vi "RTS Find Earliest Start Time.vi"(8 "Error In":errorcluster, 11 "All Door Opener Ctrl":T4 {"Station 8"."Station Slide"."Chamber 1-1"."Start Time" format="%<%X\n%x>T"; "Station 8"."Station Slide"."Chamber 1-1"."End Time" format="%<%X\n%x>T"; "Station 8"."Station Slide"."Time Count (s)" format="%.2f"; "Station 8"."Station Cab"."Chamber 1-1"."Start Time" format="%<%X\n%x>T"; "Station 8"."Station Cab"."Chamber 1-1"."End Time" format="%<%X\n%x>T"; "Station 8"."Station Cab"."Time Count (s)" format="%.2f"; "Station 8"."Station Freezer"."Chamber 1-1"."Start Time" format="%<%X\n%x>T"; "Station 8"."Station Freezer"."Chamber 1-1"."End Time" format="%<%X\n%x>T"; "Station 8"."Station Freezer"."Time Count (s)" format="%.2f"; "Station 7"."Station Slide"."Chamber 1-1"."Start Time" format="%<%X\n%x>T"; "Station 7"."Station Slide"."Chamber 1-1"."End Time" format="%<%X\n%x>T"; "Station 7"."Station Slide"."Time Count (s)" format="%.2f"; "Station 7"."Station Cab"."Chamber 1-1"."Start Time" format="%<%X\n%x>T"; "Station 7"."Station Cab"."Chamber 1-1"."End Time" format="%<%X\n%x>T"; "Station 7"."Station Cab"."Time Count (s)" format="%.2f"; "Station 7"."Station Freezer"."Chamber 1-1"."Start Time" format="%<%X\n%x>T"; "Station 7"."Station Freezer"."Chamber 1-1"."End Time" format="%<%X\n%x>T"; "Station 7"."Station Freezer"."Time Count (s)" format="%.2f"; "Station 6"."Station Slide"."Chamber 1-1"."Start Time" format="%<%X\n%x>T"; "Station 6"."Station Slide"."Chamber 1-1"."End Time" format="%<%X\n%x>T"; "Station 6"."Station Slide"."Time Count (s)" format="%.2f"; "Station 6"."Station Cab"."Chamber 1-1"."Start Time" format="%<%X\n%x>T"; "Station 6"."Station Cab"."Chamber 1-1"."End Time" format="%<%X\n%x>T"; "Station 6"."Station Cab"."Time Count (s)" format="%.2f"; "Station 6"."Station Freezer"."Chamber 1-1"."Start Time" format="%<%X\n%x>T"; "Station 6"."Station Freezer"."Chamber 1-1"."End Time" format="%<%X\n%x>T"; "Station 6"."Station Freezer"."Time Count (s)" format="%.2f"; "Station 5"."Station Slide"."Chamber 1-1"."Start Time" format="%<%X\n%x>T"; "Station 5"."Station Slide"."Chamber 1-1"."End Time" format="%<%X\n%x>T"; "Station 5"."Station Slide"."Time Count (s)" format="%.2f"; "Station 5"."Station Cab"."Chamber 1-1"."Start Time" format="%<%X\n%x>T"; "Station 5"."Station Cab"."Chamber 1-1"."End Time" format="%<%X\n%x>T"; "Station 5"."Station Cab"."Time Count (s)" format="%.2f"; "Station 5"."Station Freezer"."Chamber 1-1"."Start Time" format="%<%X\n%x>T"; "Station 5"."Station Freezer"."Chamber 1-1"."End Time" format="%<%X\n%x>T"; "Station 5"."Station Freezer"."Time Count (s)" format="%.2f"; "Station 4"."Station Slide"."Chamber 1-1"."Start Time" format="%<%X\n%x>T"; "Station 4"."Station Slide"."Chamber 1-1"."End Time" format="%<%X\n%x>T"; "Station 4"."Station Slide"."Time Count (s)" format="%.2f"; "Station 4"."Station Cab"."Chamber 1-1"."Start Time" format="%<%X\n%x>T"; "Station 4"."Station Cab"."Chamber 1-1"."End Time" format="%<%X\n%x>T"; "Station 4"."Station Cab"."Time Count (s)" format="%.2f"; "Station 4"."Station Freezer"."Chamber 1-1"."Start Time" format="%<%X\n%x>T"; "Station 4"."Station Freezer"."Chamber 1-1"."End Time" format="%<%X\n%x>T"; "Station 4"."Station Freezer"."Time Count (s)" format="%.2f"; "Station 3"."Station Slide"."Chamber 1-1"."Start Time" format="%<%X\n%x>T"; "Station 3"."Station Slide"."Chamber 1-1"."End Time" format="%<%X\n%x>T"; "Station 3"."Station Slide"."Time Count (s)" format="%.2f"; "Station 3"."Station Cab"."Chamber 1-1"."Start Time" format="%<%X\n%x>T"; "Station 3"."Station Cab"."Chamber 1-1"."End Time" format="%<%X\n%x>T"; "Station 3"."Station Cab"."Time Count (s)" format="%.2f"; "Station 3"."Station Freezer"."Chamber 1-1"."Start Time" format="%<%X\n%x>T"; "Station 3"."Station Freezer"."Chamber 1-1"."End Time" format="%<%X\n%x>T"; "Station 3"."Station Freezer"."Time Count (s)" format="%.2f"; "Station 2"."Station Slide"."Chamber 1-1"."Start Time" format="%<%X\n%x>T"; "Station 2"."Station Slide"."Chamber 1-1"."End Time" format="%<%X\n%x>T"; "Station 2"."Station Slide"."Time Count (s)" format="%.2f"; "Station 2"."Station Cab"."Chamber 1-1"."Start Time" format="%<%X\n%x>T"; "Station 2"."Station Cab"."Chamber 1-1"."End Time" format="%<%X\n%x>T"; "Station 2"."Station Cab"."Time Count (s)" format="%.2f"; "Station 2"."Station Freezer"."Chamber 1-1"."Start Time" format="%<%X\n%x>T"; "Station 2"."Station Freezer"."Chamber 1-1"."End Time" format="%<%X\n%x>T"; "Station 2"."Station Freezer"."Time Count (s)" format="%.2f"; "Station 1"."Station Slide"."Chamber 1-1"."Start Time" format="%<%X\n%x>T"; "Station 1"."Station Slide"."Chamber 1-1"."End Time" format="%<%X\n%x>T"; "Station 1"."Station Slide"."Time Count (s)" format="%.2f"; "Station 1"."Station Cab"."Chamber 1-1"."Start Time" format="%<%X\n%x>T"; "Station 1"."Station Cab"."Chamber 1-1"."End Time" format="%<%X\n%x>T"; "Station 1"."Station Cab"."Time Count (s)" format="%.2f"; "Station 1"."Station Freezer"."Chamber 1-1"."Start Time" format="%<%X\n%x>T"; "Station 1"."Station Freezer"."Chamber 1-1"."End Time" format="%<%X\n%x>T"; "Station 1"."Station Freezer"."Time Count (s)" format="%.2f"}) -> (0 "Error Out":errorcluster, 2 "Index":i32, 3 "Chamber 1-1":T1={"End Time"=timestamp(0 s since 1904-01-01), "Start Time"=timestamp(0 s since 1904-01-01), "Door Opening Schedule:"={"Open Door Timer (s)"=10.0, "Delay Time (s)"=10.0, "Close Door Timer (s)"=10.0}, "Enable Door Ops"=FALSE, "Door Openings"=0, "Temp (°F)"=0.0, "Humidity (%)"=0.0, "Voltage (V)"=0.0, "Door Open Sequence:"=enum."", "Door Delay(sec)"=0.0, "Dehum (°F)"=0.0, "Cool (°F)"=0.0} {"Start Time" format="%<%X\n%x>T"; "End Time" format="%<%X\n%x>T"})   [LabVIEW 2016]
uses:
  Type Definitions/RTS All Station Door Opener Ctrl.ctl
  Type Definitions/RTS Station Relay Ops.ctl
  Type Definitions/RTS Door Opener Indicator.ctl
  Type Definitions/RTS Door Ops Client.ctl
  Type Definitions/RTS Door Opening Schedule.ctl
  Type Definitions/RTS Door Ops Sequence.ctl
panel:
  # "Chamber Conditions:"
  # "Chamber Conditions:"
  # "Chamber Conditions:"
  # "Chamber Conditions:"
  # "Chamber Conditions:"
  # "Chamber Conditions:"
  # "Chamber Conditions:"
  # "Chamber Conditions:"
  # "Chamber Conditions:"
  # "Chamber Conditions:"
  # "Chamber Conditions:"
  # "Chamber Conditions:"
  # "Chamber Conditions:"
  # "Chamber Conditions:"
  # "Chamber Conditions:"
  # "Chamber Conditions:"
  # "Chamber Conditions:"
  # "Chamber Conditions:"
  # "Chamber Conditions:"
  # "Chamber Conditions:"
  # "Chamber Conditions:"
  # "Chamber Conditions:"
  # "Chamber Conditions:"
  # "Chamber Conditions:"
  # "Chamber Conditions:"
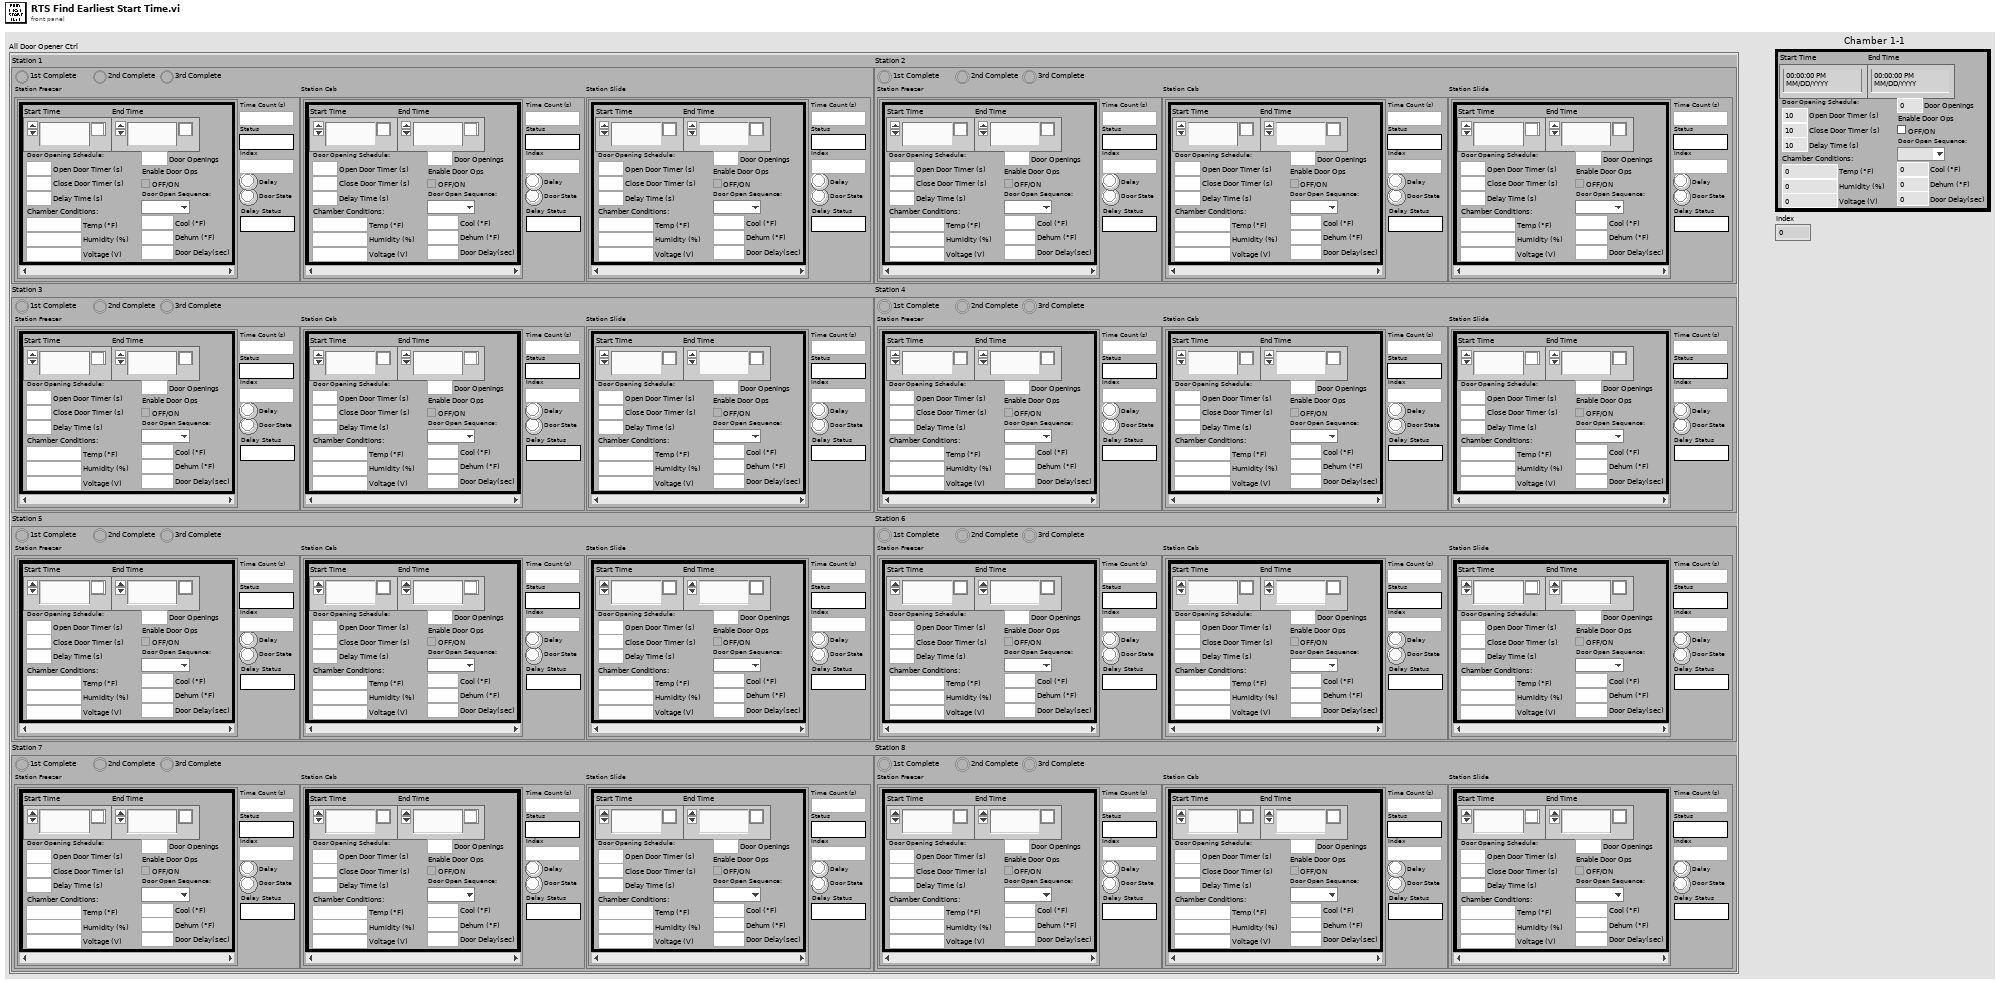
[diagram p1: front panel]
types:
  T1 = typedef "RTS Door Ops Client.ctl" = cluster{"End Time":timestamp, "Start Time":timestamp, "Door Opening Schedule:":T2, "Enable Door Ops":bool, "Door Openings":u32, "Temp (°F)":dbl, "Humidity (%)":dbl, "Voltage (V)":dbl, "Door Open Sequence:":T3, "Door Delay(sec)":dbl, "Dehum (°F)":dbl, "Cool (°F)":dbl}
  T2 = typedef "RTS Door Opening Schedule.ctl" = cluster{"Open Door Timer (s)":dbl, "Delay Time (s)":dbl, "Close Door Timer (s)":dbl}
  T3 = typedef "RTS Door Ops Sequence.ctl" = enum16{"", "1st", "2nd", "3rd"}
  T4 = typedef "RTS All Station Door Opener Ctrl.ctl" = cluster{"Station 1":T5, "Station 2":T5, "Station 3":T5, "Station 4":T5, "Station 5":T5, "Station 6":T5, "Station 7":T5, "Station 8":T5}
  T5 = typedef "RTS Station Relay Ops.ctl" = cluster{"Station Freezer":T6, "Station Cab":T6, "Station Slide":T6, "1st Complete":bool, "2nd Complete":bool, "3rd Complete":bool}
  T6 = typedef "RTS Door Opener Indicator.ctl" = cluster{"Time Count (s)":dbl, "Status":string, "Door State":bool, "Delay":bool, "Chamber 1-1":T1[], "Index":i32, "Delay Status":string}
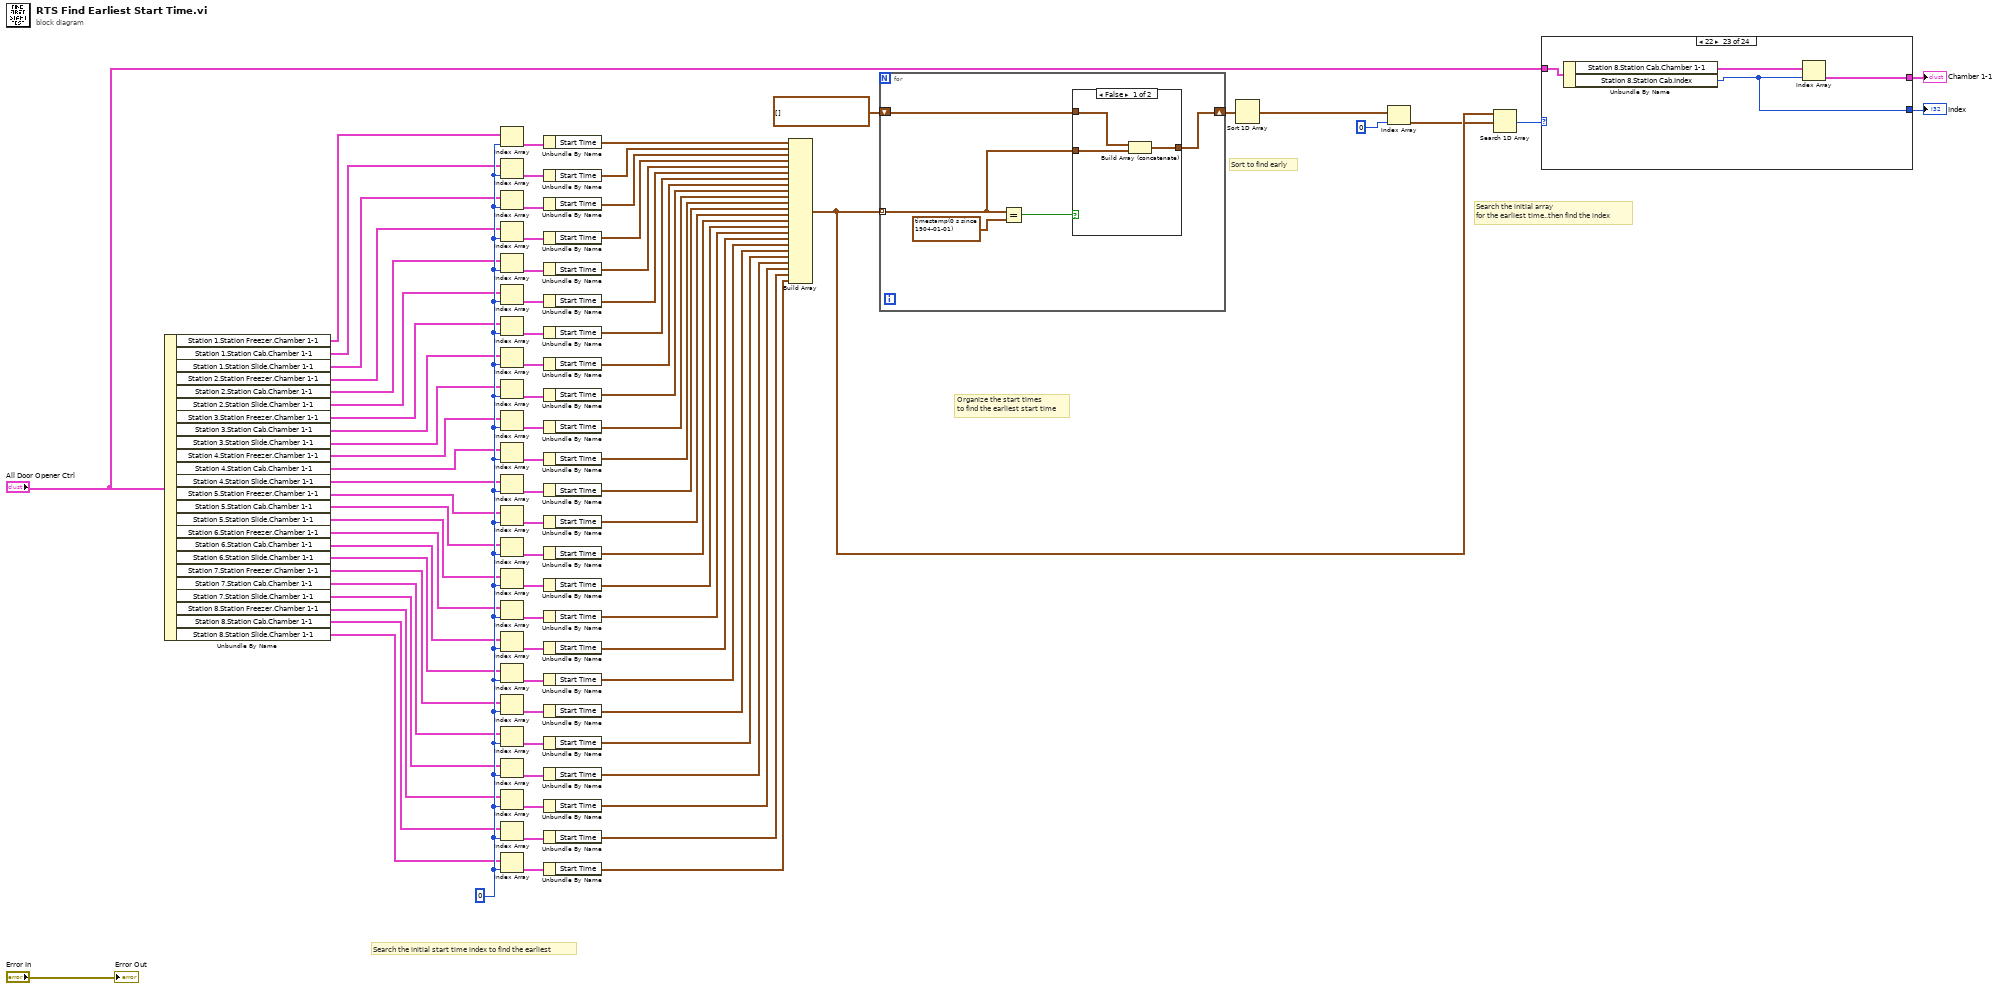
[diagram p0: block diagram]
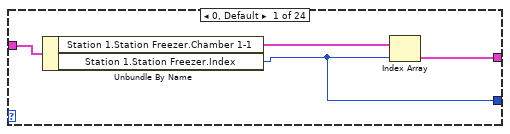
[diagram p2: hidden frame]
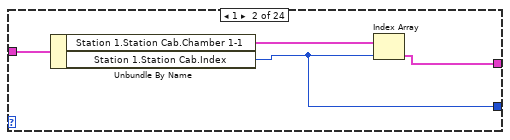
[diagram p3: hidden frame]
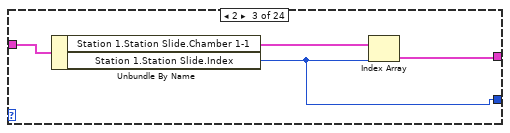
[diagram p4: hidden frame]
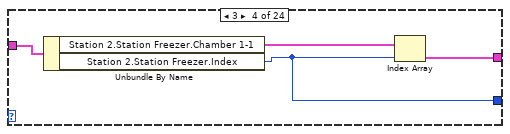
[diagram p5: hidden frame]
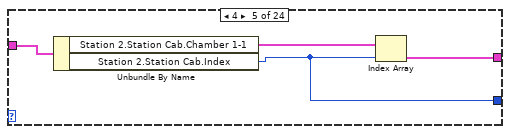
[diagram p6: hidden frame]
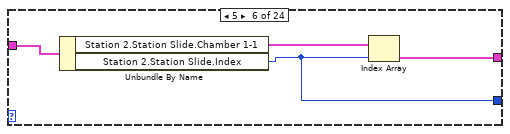
[diagram p7: hidden frame]
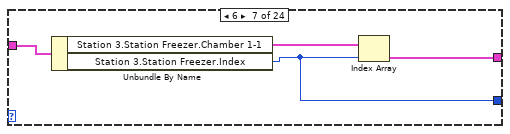
[diagram p8: hidden frame]
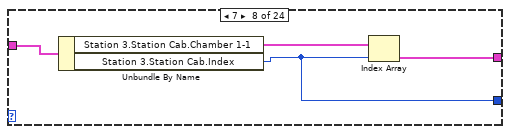
[diagram p9: hidden frame]
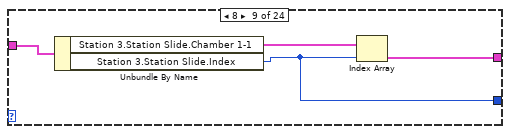
[diagram p10: hidden frame]
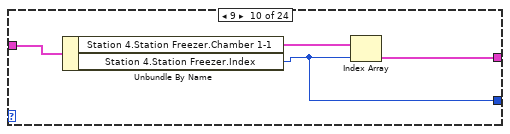
[diagram p11: hidden frame]
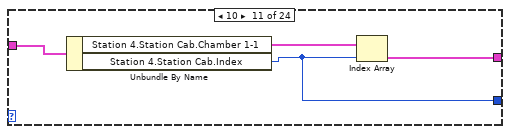
[diagram p12: hidden frame]
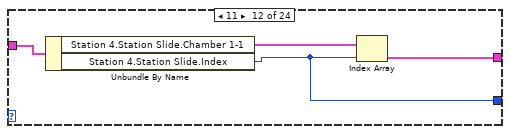
[diagram p13: hidden frame]
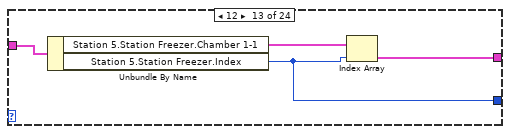
[diagram p14: hidden frame]
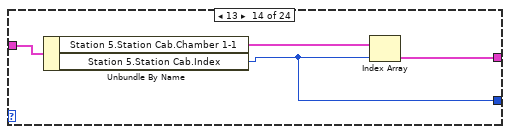
[diagram p15: hidden frame]
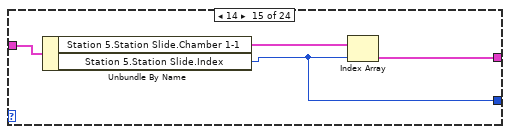
[diagram p16: hidden frame]
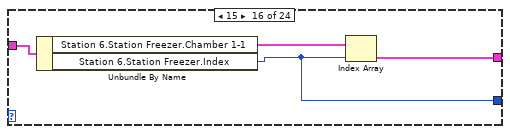
[diagram p17: hidden frame]
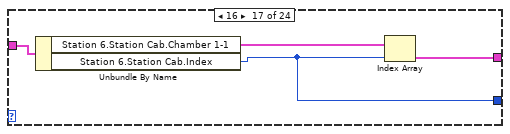
[diagram p18: hidden frame]
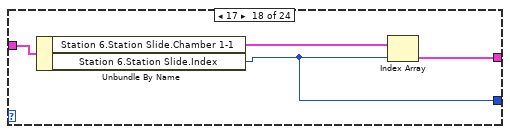
[diagram p19: hidden frame]
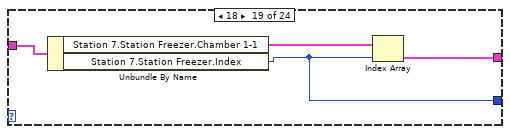
[diagram p20: hidden frame]
diagram:
  w36 = 0 ("index")
  # "Sort to find early"
  # "Search the initial start time index to find the earliest"
  # "Search the initial array\nfor the earliest time..then find the index"
  # "Organize the start times \nto find the earliest start time"
  n1 = Unbundle By Name("All Door Opener Ctrl") -> ("Station 1.Station Freezer.Chamber 1-1"=w35:T1[], "Station 1.Station Cab.Chamber 1-1"=w34:T1[], "Station 1.Station Slide.Chamber 1-1"=w33:T1[], "Station 2.Station Freezer.Chamber 1-1"=w32:T1[], "Station 2.Station Cab.Chamber 1-1"=w31:T1[], "Station 2.Station Slide.Chamber 1-1"=w30:T1[], "Station 3.Station Freezer.Chamber 1-1"=w29:T1[], "Station 3.Station Cab.Chamber 1-1"=w28:T1[], "Station 3.Station Slide.Chamber 1-1"=w27:T1[], "Station 4.Station Freezer.Chamber 1-1"=w26:T1[], "Station 4.Station Cab.Chamber 1-1"=w25:T1[], "Station 4.Station Slide.Chamber 1-1"=w24:T1[], "Station 5.Station Freezer.Chamber 1-1"=w23:T1[], "Station 5.Station Cab.Chamber 1-1"=w22:T1[], "Station 5.Station Slide.Chamber 1-1"=w21:T1[], "Station 6.Station Freezer.Chamber 1-1"=w20:T1[], "Station 6.Station Cab.Chamber 1-1"=w19:T1[], "Station 6.Station Slide.Chamber 1-1"=w18:T1[], "Station 7.Station Freezer.Chamber 1-1"=w17:T1[], "Station 7.Station Cab.Chamber 1-1"=w16:T1[], "Station 7.Station Slide.Chamber 1-1"=w15:T1[], "Station 8.Station Freezer.Chamber 1-1"=w14:T1[], "Station 8.Station Cab.Chamber 1-1"=w13:T1[], "Station 8.Station Slide.Chamber 1-1"=w12:T1[])
  n2 = Index Array(array=w35, index=w36) -> (element=w37:T1)
  n3 = Index Array(array=w34, index=w36) -> (element=w38:T1)
  n4 = Index Array(array=w33, index=w36) -> (element=w39:T1)
  n5 = Index Array(array=w32, index=w36) -> (element=w40:T1)
  n6 = Index Array(array=w31, index=w36) -> (element=w41:T1)
  n7 = Index Array(array=w30, index=w36) -> (element=w42:T1)
  n8 = Index Array(array=w29, index=w36) -> (element=w43:T1)
  n9 = Index Array(array=w28, index=w36) -> (element=w44:T1)
  n10 = Index Array(array=w27, index=w36) -> (element=w45:T1)
  n11 = Index Array(array=w26, index=w36) -> (element=w46:T1)
  n12 = Index Array(array=w25, index=w36) -> (element=w47:T1)
  n13 = Index Array(array=w24, index=w36) -> (element=w48:T1)
  n14 = Index Array(array=w23, index=w36) -> (element=w49:T1)
  n15 = Index Array(array=w22, index=w36) -> (element=w50:T1)
  n16 = Index Array(array=w21, index=w36) -> (element=w51:T1)
  n17 = Index Array(array=w20, index=w36) -> (element=w52:T1)
  n18 = Index Array(array=w19, index=w36) -> (element=w53:T1)
  n19 = Index Array(array=w18, index=w36) -> (element=w54:T1)
  n20 = Index Array(array=w17, index=w36) -> (element=w55:T1)
  n21 = Index Array(array=w16, index=w36) -> (element=w56:T1)
  n22 = Index Array(array=w15, index=w36) -> (element=w57:T1)
  n23 = Index Array(array=w14, index=w36) -> (element=w58:T1)
  n24 = Index Array(array=w13, index=w36) -> (element=w59:T1)
  n25 = Index Array(array=w12, index=w36) -> (element=w60:T1)
  n26 = Unbundle By Name(w37) -> ("Start Time"=w61:timestamp)
  n27 = Unbundle By Name(w38) -> ("Start Time"=w62:timestamp)
  n28 = Unbundle By Name(w39) -> ("Start Time"=w63:timestamp)
  n29 = Unbundle By Name(w40) -> ("Start Time"=w64:timestamp)
  n30 = Unbundle By Name(w41) -> ("Start Time"=w65:timestamp)
  n31 = Unbundle By Name(w42) -> ("Start Time"=w66:timestamp)
  n32 = Unbundle By Name(w43) -> ("Start Time"=w67:timestamp)
  n33 = Unbundle By Name(w44) -> ("Start Time"=w68:timestamp)
  n34 = Unbundle By Name(w45) -> ("Start Time"=w69:timestamp)
  n35 = Unbundle By Name(w46) -> ("Start Time"=w70:timestamp)
  n36 = Unbundle By Name(w47) -> ("Start Time"=w71:timestamp)
  n37 = Unbundle By Name(w48) -> ("Start Time"=w72:timestamp)
  n38 = Unbundle By Name(w49) -> ("Start Time"=w73:timestamp)
  n39 = Unbundle By Name(w50) -> ("Start Time"=w74:timestamp)
  n40 = Unbundle By Name(w51) -> ("Start Time"=w75:timestamp)
  n41 = Unbundle By Name(w52) -> ("Start Time"=w76:timestamp)
  n42 = Unbundle By Name(w53) -> ("Start Time"=w77:timestamp)
  n43 = Unbundle By Name(w54) -> ("Start Time"=w78:timestamp)
  n44 = Unbundle By Name(w55) -> ("Start Time"=w79:timestamp)
  n45 = Unbundle By Name(w56) -> ("Start Time"=w80:timestamp)
  n46 = Unbundle By Name(w57) -> ("Start Time"=w81:timestamp)
  n47 = Unbundle By Name(w58) -> ("Start Time"=w82:timestamp)
  n48 = Unbundle By Name(w59) -> ("Start Time"=w83:timestamp)
  n49 = Unbundle By Name(w60) -> ("Start Time"=w84:timestamp)
  n50 = Build Array(w61, w62, w63, w64, w65, w66, w67, w68, w69, w70, w71, w72, w73, w74, w75, w76, w77, w78, w79, w80, w81, w82, w83, w84) -> (w7:timestamp[])
  n51 = for {
    tunnel: w7 -> [w86] mode=indexing
    shift-right: [w87] -> w9
    shift-left: timestamp[] [] -> [w88]
    n52 = Equal?(x=w86, y=timestamp(0 s since 1904-01-01)) -> (x = y?=w85:bool)
    n53 = case shown="False" w85 {
      tunnel: w86 -> [w92 _]
      tunnel: w88 -> [w91 w93]
      tunnel: [w90 w93] -> w87
      frame False {
        n54 = Build Array (concatenate)(w91, w92) -> (w90:timestamp[])
      }
      frame True {
      }
    }
  }
  n55 = Sort 1D Array(array=w9) -> (sorted array=w1:timestamp[])
  n56 = Index Array(array=w1, index=0) -> (element=w6:timestamp)
  n57 = Search 1D Array(1D array=w7, element=w6) -> (index of element=w4:i32)  [unwired: 1 in]
  n58 = case shown="22" w4 {
    tunnel: "All Door Opener Ctrl" -> [w97 w101 w105 w109 w113 w117 w121 w125 w129 w133 w137 w141 w145 w149 w153 w157 w161 w165 w169 w173 w177 w181 w185 w189]
    tunnel: [w95 w99 w103 w107 w111 w115 w119 w123 w127 w131 w135 w139 w143 w147 w151 w155 w159 w163 w167 w171 w175 w179 w183 w187] -> w2
    tunnel: [w94 w98 w102 w106 w110 w114 w118 w122 w126 w130 w134 w138 w142 w146 w150 w154 w158 w162 w166 w170 w174 w178 w182 w186] -> w3
    frame 0, Default {
      n59 = Unbundle By Name(w97) -> ("Station 1.Station Freezer.Chamber 1-1"=w96:T1[], "Station 1.Station Freezer.Index"=w94:i32)
      n60 = Index Array(array=w96, index=w94) -> (element=w95:T1)
    }
    frame 1 {
      n61 = Unbundle By Name(w101) -> ("Station 1.Station Cab.Chamber 1-1"=w100:T1[], "Station 1.Station Cab.Index"=w98:i32)
      n62 = Index Array(array=w100, index=w98) -> (element=w99:T1)
    }
    frame 2 {
      n63 = Unbundle By Name(w105) -> ("Station 1.Station Slide.Chamber 1-1"=w104:T1[], "Station 1.Station Slide.Index"=w102:i32)
      n64 = Index Array(array=w104, index=w102) -> (element=w103:T1)
    }
    frame 3 {
      n65 = Unbundle By Name(w109) -> ("Station 2.Station Freezer.Chamber 1-1"=w108:T1[], "Station 2.Station Freezer.Index"=w106:i32)
      n66 = Index Array(array=w108, index=w106) -> (element=w107:T1)
    }
    frame 4 {
      n67 = Unbundle By Name(w113) -> ("Station 2.Station Cab.Chamber 1-1"=w112:T1[], "Station 2.Station Cab.Index"=w110:i32)
      n68 = Index Array(array=w112, index=w110) -> (element=w111:T1)
    }
    frame 5 {
      n69 = Unbundle By Name(w117) -> ("Station 2.Station Slide.Chamber 1-1"=w116:T1[], "Station 2.Station Slide.Index"=w114:i32)
      n70 = Index Array(array=w116, index=w114) -> (element=w115:T1)
    }
    frame 6 {
      n71 = Unbundle By Name(w121) -> ("Station 3.Station Freezer.Chamber 1-1"=w120:T1[], "Station 3.Station Freezer.Index"=w118:i32)
      n72 = Index Array(array=w120, index=w118) -> (element=w119:T1)
    }
    frame 7 {
      n73 = Unbundle By Name(w125) -> ("Station 3.Station Cab.Chamber 1-1"=w124:T1[], "Station 3.Station Cab.Index"=w122:i32)
      n74 = Index Array(array=w124, index=w122) -> (element=w123:T1)
    }
    frame 8 {
      n75 = Unbundle By Name(w129) -> ("Station 3.Station Slide.Chamber 1-1"=w128:T1[], "Station 3.Station Slide.Index"=w126:i32)
      n76 = Index Array(array=w128, index=w126) -> (element=w127:T1)
    }
    frame 9 {
      n77 = Unbundle By Name(w133) -> ("Station 4.Station Freezer.Chamber 1-1"=w132:T1[], "Station 4.Station Freezer.Index"=w130:i32)
      n78 = Index Array(array=w132, index=w130) -> (element=w131:T1)
    }
    frame 10 {
      n79 = Unbundle By Name(w137) -> ("Station 4.Station Cab.Chamber 1-1"=w136:T1[], "Station 4.Station Cab.Index"=w134:i32)
      n80 = Index Array(array=w136, index=w134) -> (element=w135:T1)
    }
    frame 11 {
      n81 = Unbundle By Name(w141) -> ("Station 4.Station Slide.Chamber 1-1"=w140:T1[], "Station 4.Station Slide.Index"=w138:i32)
      n82 = Index Array(array=w140, index=w138) -> (element=w139:T1)
    }
    frame 12 {
      n83 = Unbundle By Name(w145) -> ("Station 5.Station Freezer.Chamber 1-1"=w144:T1[], "Station 5.Station Freezer.Index"=w142:i32)
      n84 = Index Array(array=w144, index=w142) -> (element=w143:T1)
    }
    frame 13 {
      n85 = Unbundle By Name(w149) -> ("Station 5.Station Cab.Chamber 1-1"=w148:T1[], "Station 5.Station Cab.Index"=w146:i32)
      n86 = Index Array(array=w148, index=w146) -> (element=w147:T1)
    }
    frame 14 {
      n87 = Unbundle By Name(w153) -> ("Station 5.Station Slide.Chamber 1-1"=w152:T1[], "Station 5.Station Slide.Index"=w150:i32)
      n88 = Index Array(array=w152, index=w150) -> (element=w151:T1)
    }
    frame 15 {
      n89 = Unbundle By Name(w157) -> ("Station 6.Station Freezer.Chamber 1-1"=w156:T1[], "Station 6.Station Freezer.Index"=w154:i32)
      n90 = Index Array(array=w156, index=w154) -> (element=w155:T1)
    }
    frame 16 {
      n91 = Unbundle By Name(w161) -> ("Station 6.Station Cab.Chamber 1-1"=w160:T1[], "Station 6.Station Cab.Index"=w158:i32)
      n92 = Index Array(array=w160, index=w158) -> (element=w159:T1)
    }
    frame 17 {
      n93 = Unbundle By Name(w165) -> ("Station 6.Station Slide.Chamber 1-1"=w164:T1[], "Station 6.Station Slide.Index"=w162:i32)
      n94 = Index Array(array=w164, index=w162) -> (element=w163:T1)
    }
    frame 18 {
      n95 = Unbundle By Name(w169) -> ("Station 7.Station Freezer.Chamber 1-1"=w168:T1[], "Station 7.Station Freezer.Index"=w166:i32)
      n96 = Index Array(array=w168, index=w166) -> (element=w167:T1)
    }
    frame 19 {
      n97 = Unbundle By Name(w173) -> ("Station 7.Station Cab.Chamber 1-1"=w172:T1[], "Station 7.Station Cab.Index"=w170:i32)
      n98 = Index Array(array=w172, index=w170) -> (element=w171:T1)
    }
    frame 20 {
      n99 = Unbundle By Name(w177) -> ("Station 7.Station Slide.Chamber 1-1"=w176:T1[], "Station 7.Station Slide.Index"=w174:i32)
      n100 = Index Array(array=w176, index=w174) -> (element=w175:T1)
    }
    frame 21 {
      n101 = Unbundle By Name(w181) -> ("Station 8.Station Freezer.Chamber 1-1"=w180:T1[], "Station 8.Station Freezer.Index"=w178:i32)
      n102 = Index Array(array=w180, index=w178) -> (element=w179:T1)
    }
    frame 22 {
      n103 = Unbundle By Name(w185) -> ("Station 8.Station Cab.Chamber 1-1"=w184:T1[], "Station 8.Station Cab.Index"=w182:i32)
      n104 = Index Array(array=w184, index=w182) -> (element=w183:T1)
    }
    frame 23 {
      n105 = Unbundle By Name(w189) -> ("Station 8.Station Slide.Chamber 1-1"=w188:T1[], "Station 8.Station Slide.Index"=w186:i32)
      n106 = Index Array(array=w188, index=w186) -> (element=w187:T1)
    }
  }
  "Index" <- w3
  "Chamber 1-1" <- w2
  "Error Out" <- "Error In"
